vi "globalTearDown.vi"(8 "error in (no error)":errorcluster, 11 "Single Core Simple Loopback in":refnum<class "Octal Loopback.lvclass">) -> (0 "error out":errorcluster, 3 "Single Core Simple Loopback out":refnum<class "Octal Loopback.lvclass">)   [LabVIEW 2020, in "Octal Loopback.lvclass"]
uses:
  Octal Loopback.lvclass
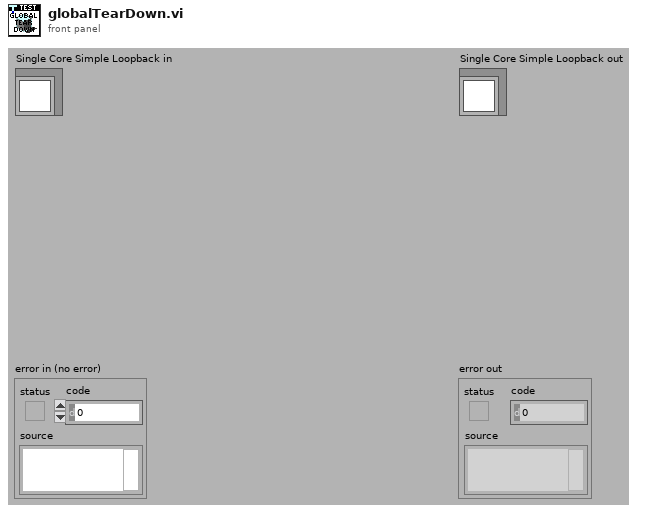
[diagram p1: front panel]
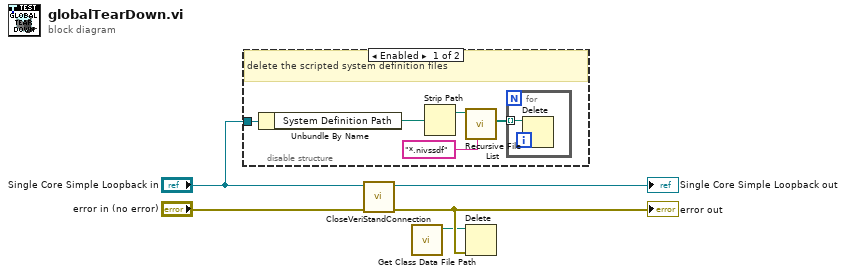
[diagram p0: block diagram]
diagram:
  n1 = disable-structure shown="Enabled" {
    disable-tunnel: "Single Core Simple Loopback in" -> [w10 _]
    frame Enabled {
      # "delete the scripted system definition files"
      n2 = Unbundle By Name(w10) -> ("System Definition Path"=w7:path)
      n3 = Strip Path(path=w7) -> (stripped path=w6:path)  [unwired: 1 out]
      n4 = call <vilib>:"Recursive File List.vi"("pattern"="*.nivssdf", "Folder Path"=w6) -> ("All Files in Dir"=w8:path[])  [unwired: 5 in, 4 out]
      n5 = for {
        tunnel: w8 -> [w11] mode=indexing
        n6 = Delete(path (use dialog)=w11) -> ()  [unwired: 4 in, 3 out]
      }
    }
    frame Disabled {
    }
  }
  n7 = call-dynamic "CloseVeriStandConnection.vi"("error in (no error)"="error in (no error)", "VeriStand Test Case in"="Single Core Simple Loopback in") -> ("error out"=w2:errorcluster, "VeriStand Test Case out"=→"Single Core Simple Loopback out":refnum<class "Octal Loopback.lvclass">)  [unwired: 8 in]
  "error out" <- w2
  n8 = call "Get Class Data File Path.vi"() -> ("Class Data File Path"=w1:path)  [unwired: 11 in]
  n9 = Delete(path (use dialog)=w1, error in=w2) -> ()  [unwired: 3 in, 3 out]
